vi "FCME.vi"(8 "PFA":dbl=0.01 format="%#_13g", 11 "Mag":dbl[](array[numeric])) -> (0 "Noise Floor":dbl, 3 "Threshold":dbl)   [LabVIEW 2019]
uses:
  <vilib>/Analysis/NI_AALBase.lvlib
  <vilib>/Analysis/baseanly.llb/Mean (DBL).vi
panel:
  out "Array":dbl[](array[numeric])
  in  "Iterations":i32=5
  in  "Sample Length":i32=10
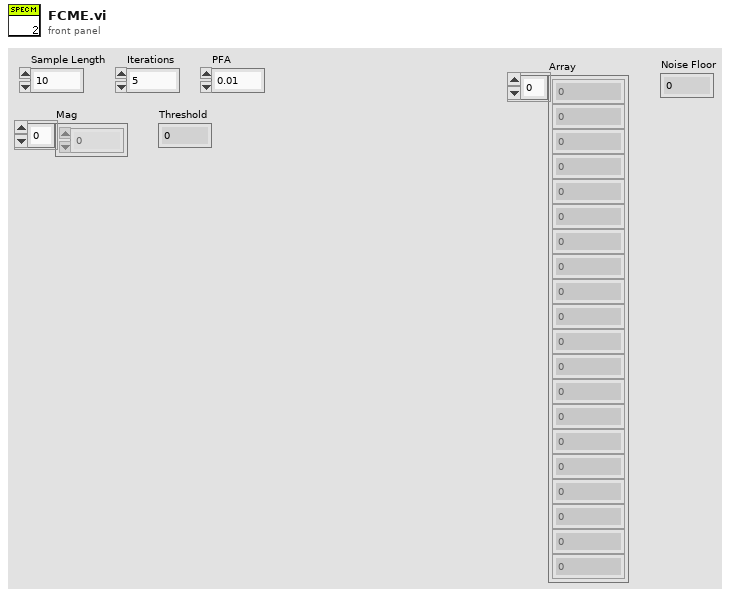
[diagram p1: front panel]
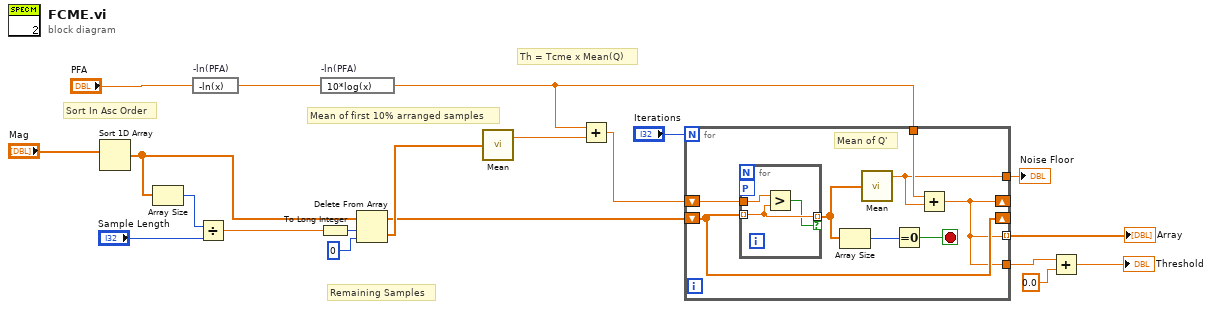
[diagram p0: block diagram]
diagram:
  # "Mean of first 10% arranged samples"
  # "Remaining Samples"
  # "Sort In Asc Order"
  # "Th = Tcme x Mean(Q)"
  n1 = Sort 1D Array(array="Mag") -> (sorted array=w12:dbl[])
  n2 = Array Size(array=w12) -> (size(s)=w6:i32)
  n3 = expression code="-ln(x)" "-ln(PFA)"("PFA") -> (w15:dbl)
  n4 = Divide(x=w6, y="Sample Length") -> (x/y=w9:dbl)
  n5 = To Long Integer(number=w9) -> (32bit integer=w18:i32)
  n6 = expression code="10*log(x)" "-ln(PFA)"(w15) -> (w16:dbl)
  n7 = Delete From Array(array=w12, length=w18, index=0) -> (deleted portion=w17:dbl[], array with subset deleted=w11:dbl[])
  n8 = call-poly <vilib>:"Mean.vi"("X"=w17) -> ("mean"=w7:dbl)  [unwired: 1 out]
  n9 = Add(x=w16, y=w7) -> (x+y=w13:dbl)
  n10 = for {
    N: "Iterations" -> [_]
    tunnel: w16 -> [w28]
    shift-right: [w21] -> _
    shift-left: w13 -> [w25]
    shift-right: [w23] -> _
    shift-left: w11 -> [w23]
    tunnel: [w21] -> w19
    tunnel: [w22] -> w4
    tunnel: [w21] -> w3 mode=indexing
    stop <- w26 stop-if-true
    # "Mean of Q'"
    n11 = for {
      tunnel: w25 -> [w31]
      tunnel: w23 -> [w30] mode=indexing
      tunnel: [w30] -> w24 mode=indexing if=w29
      workers-P: _ -> [_]
      n12 = Greater?(x=w31, y=w30) -> (0:w29:bool)
    }
    n13 = Array Size(array=w24) -> (size(s)=w27:i32)
    n14 = call-poly <vilib>:"Mean.vi"("X"=w24) -> ("mean"=w22:dbl)  [unwired: 1 out]
    n15 = Equal To 0?(x=w27) -> (x = 0?=w26:bool)
    n16 = Add(x=w28, y=w22) -> (x+y=w21:dbl)
  }
  "Noise Floor" <- w4
  "Array" <- w3
  n17 = Add(x=w19, y=0.0 ("x")) -> (x+y=→"Threshold":dbl)
